vi "proceso2.vi"() -> ()   [LabVIEW 2020]
panel:
  out "proceso 2":T1
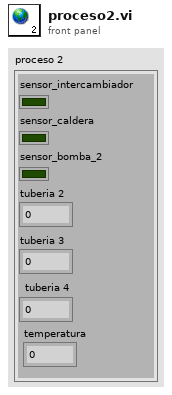
[diagram p1: front panel]
types:
  T1 = cluster{"sensor_intercambiador":bool, "sensor_caldera":bool, "sensor_bomba_2 ":bool, "tuberia 2":u8, "tuberia 3":u8, "tuberia 4":u8, "temperatura":dbl}
diagram:
